vi "zad_5_a.vi"() -> ()   [LabVIEW 2025]
uses:
  <vilib>/numeric/Random Number (Range) DBL.vi
panel:
  out "error out":errorcluster
  in  "error in":errorcluster
types:
  T1 = enum16{"open", "replace", "create", "open or create", "replace or create", "replace or create with confirmation"}
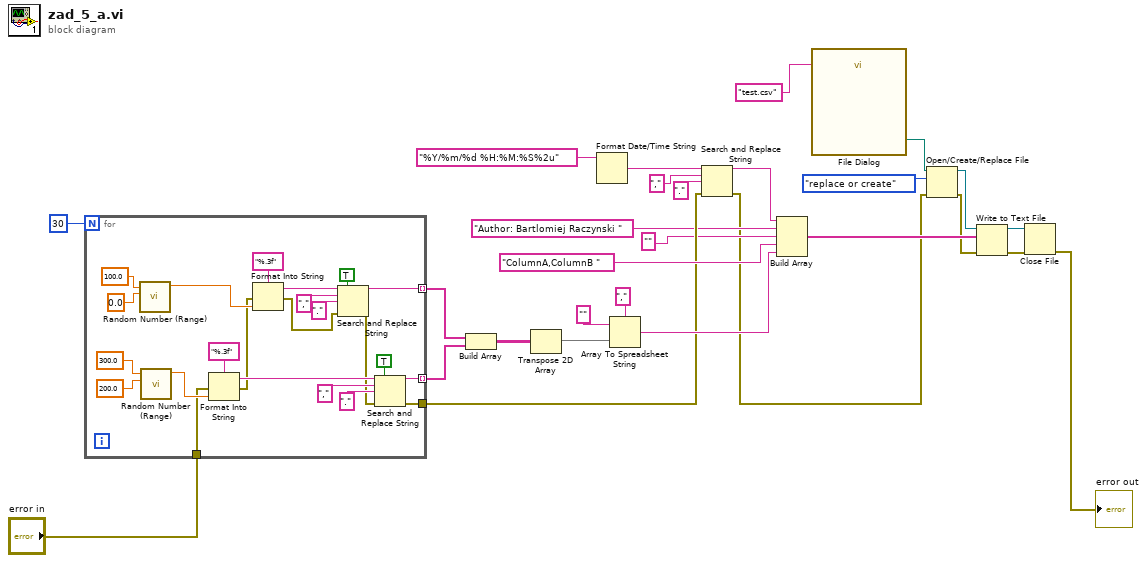
[diagram p0: block diagram]
diagram:
  n1 = for {
    N: 30 -> [_]
    tunnel: [w42] -> w20 mode=indexing
    tunnel: [w36] -> w21 mode=indexing
    tunnel: "error in" -> [w35]
    tunnel: [w29] -> w14
    n2 = call-poly <vilib>:"Random Number (Range).vi"("lower bound (0)"=0.0, "upper bound (100)"=100.0) -> ("number"=w47:dbl)  [unwired: 9 in]
    n3 = call-poly <vilib>:"Random Number (Range).vi"("lower bound (0)"=200.0, "upper bound (100)"=300.0) -> ("number"=w44:dbl)  [unwired: 9 in]
    n4 = Format Into String(format string="%.3f", error in=w35, w44) -> (resulting string=w37:string, error out=w34:errorcluster)  [unwired: 1 in]
    n5 = Format Into String(format string="%.3f", error in=w34, w47) -> (resulting string=w43:string, error out=w33:errorcluster)  [unwired: 1 in]
    n6 = Search and Replace String(replace all?=TRUE ("replace all? (F)"), input string=w43, search string=",", replace string="." ("replace string (\"\")"), error in=w33) -> (result string=w42:string, error out=w30:errorcluster)  [unwired: 3 in, 2 out]
    n7 = Search and Replace String(replace all?=TRUE ("replace all? (F)"), input string=w37, search string=",", replace string="." ("replace string (\"\")"), error in=w30) -> (result string=w36:string, error out=w29:errorcluster)  [unwired: 3 in, 2 out]
  }
  n8 = Build Array(w20, w21) -> (w23:string[][])
  n9 = Transpose 2D Array(2D array=w23) -> (transposed array=w22:string[][])
  n10 = Format Date/Time String(time format string (%c)="%Y/%m/%d %H:%M:%S%2u") -> (date/time string=w16:string)  [unwired: 2 in]
  n11 = Array To Spreadsheet String(delimiter (Tab)=",", array=w22, 3:"" ("format string")) -> (spreadsheet string=w24:string)
  n12 = Search and Replace String(input string=w16, search string=",", replace string="." ("replace string (\"\")"), error in=w14) -> (result string=w13:string, error out=w2:errorcluster)  [unwired: 4 in, 2 out]
  n13 = Build Array(w13, "Author: Bartlomiej Raczynski ", "" ("element"), "ColumnA,ColumnB ", w24) -> (w7:string[])
  n14 = call "File Dialog"("default name"="test.csv" ("pattern (all files)")) -> ("selected path"=w5:path)  [unwired: 11 in, 3 out]
  n15 = Open/Create/Replace File(file path (use dialog)=w5, error in=w2, operation (0:open)=T1."replace or create") -> (refnum out=w6:refnum<file>, error out=w3:errorcluster)  [unwired: 3 in, 1 out]
  n16 = Write to Text File(file (use dialog)=w6, text=w7, error in=w3) -> (refnum out=w8:refnum<file>, error out=w10:errorcluster)  [unwired: 1 in, 1 out]
  n17 = Close File(refnum=w8, error in=w10) -> (error out=→"error out":errorcluster)  [unwired: 1 out]
